vi "Untitled 2.vi"() -> ()   [LabVIEW 2019]
uses:
  <vilib>/OPCUA/controls/OPC UA Client Refnum.ctl
  subVIs/Mode-Ctrl.ctl
  subVIs/CMD-Ctrl.ctl
  <vilib>/OPCUA/controls/Write Variant Request.ctl
  <vilib>/OPCUA/controls/NodeId.ctl
  <vilib>/OPCUA/controls/Write Status.ctl
  <vilib>/OPCUA/client/Multiple Write Variant.vi
  <vilib>/OPCUA/NI OPC UA Client.lvlib
panel:
  out "Control Mode 5":T1
  out "Control Mode 4":T1
  out "Control Mode 3":T1
  out "Control Mode 2":T1
  out "Control Mode":T1
  in  "Reset Alarms UT":bool
  in  "Reset Commands UT":bool
  out "?":T2
  out "?":T2
  in  "Reset Alarms Tube":bool
  in  "Reset Commands Tube":bool
  out "?":T2
  out "?":T2
  in  "Reset Alarms Fork":bool
  in  "Reset Commands Fork":bool
  out "?":T2
  out "?":T2
  in  "Reset Alarms Main2":bool
  in  "Reset Commands Main2":bool
  out "?":T2
  out "?":T2
  in  "Reset Alarms Main1":bool
  in  "Reset Commands Main1":bool
  out "?":T2
  out "?":T2
  in  "error IO":errorcluster
  in  "OPC UA client refnum out":T3
  in  "stop":bool
  # "Main 1"
  # "Main 2"
  # "Fork"
  # "Tube"
  # "UT"
  # "Telescope ShutDown Command"
  # "Alt ShutDown Command"
  # "Az ShutDown Command"
  # "HSB ShutDown Command"
  # "Rotator ShutDown Command"
  # "Adaptor ShutDown Command"
  # "Enclosure ShutDown Command"
  # "MirrorCover ShutDown Command"
  # "Balancin ShutDown Command"
  # "M2 ShutDown Command"
  # "Instrument ShutDown Command"
  # "Control Mode"
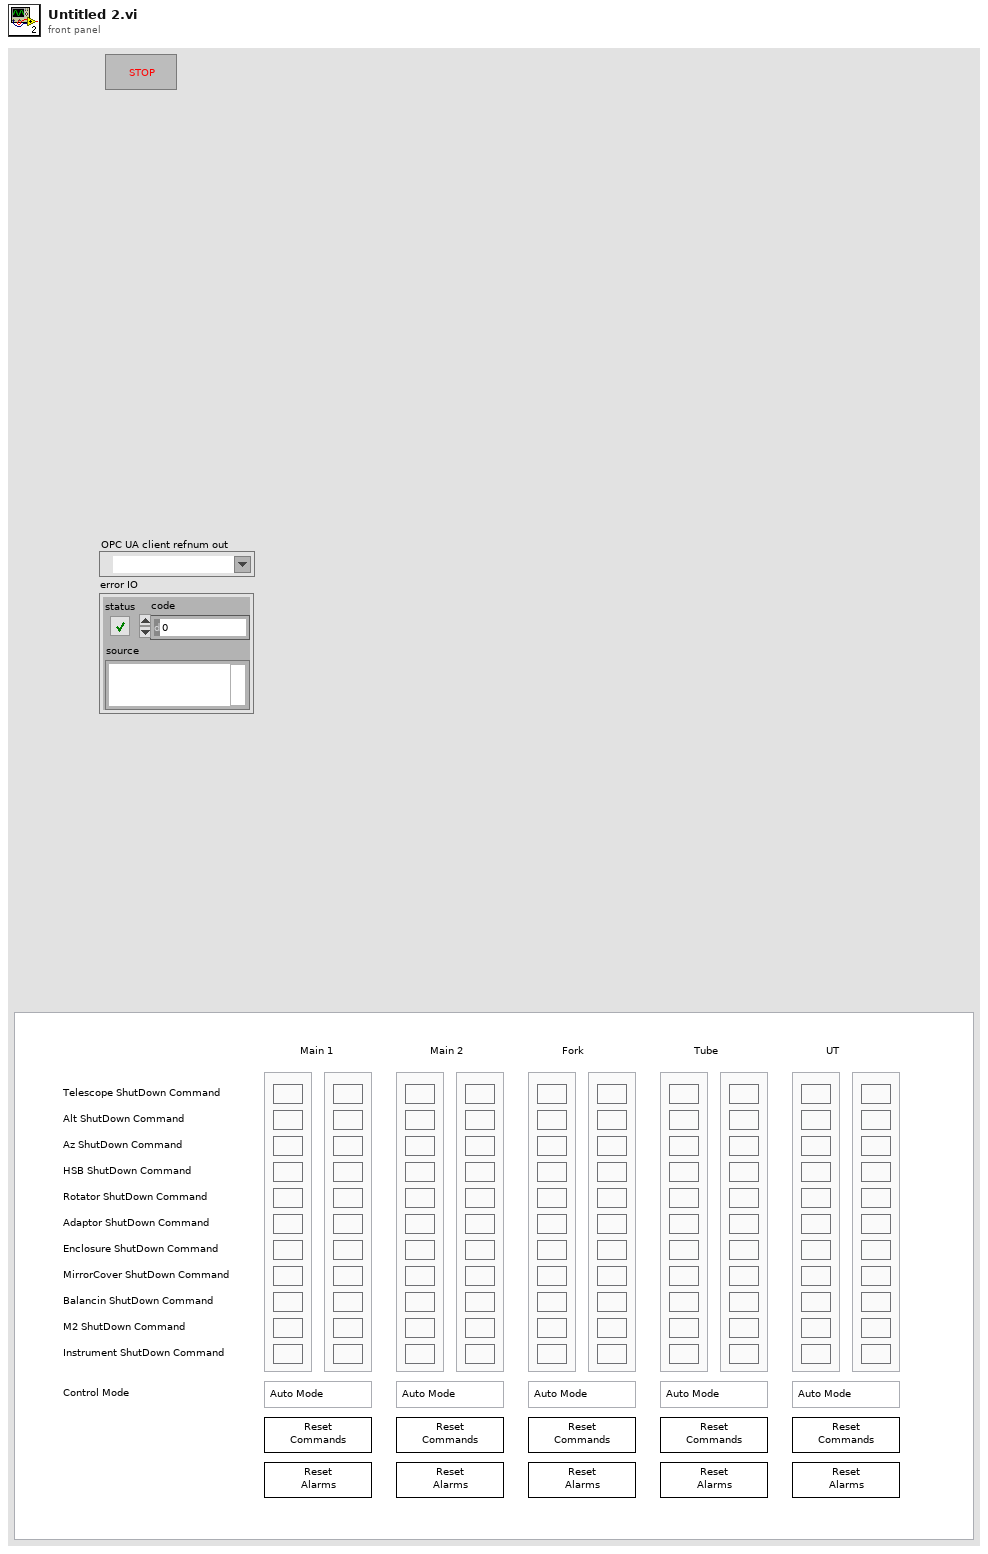
[diagram p1: front panel]
types:
  T1 = typedef "Mode-Ctrl.ctl" = enum16{"Auto Mode", "Maintenance Full Access", "Engineering Mode"}
  T2 = typedef "CMD-Ctrl.ctl" = cluster{"Telescope ShutDown Command":bool, "Alt ShutDown Command":bool, "Az ShutDown Command":bool, "HSB ShutDown Command":bool, "Rotator ShutDown Command":bool, "Adaptor ShutDown Command":bool, "Enclosure ShutDown Command":bool, "MirrorCover ShutDown Command":bool, "Balancing ShutDown Command":bool, "M2 ShutDown Command":bool, "Instrument ShutDown Command":bool}
  T3 = typedef "OPC UA Client Refnum.ctl" = refnum<k21>
  T4 = typedef "Write Variant Request.ctl" = cluster{"node ID":T5, "value":variant, "timestamp (current time)":timestamp, "node status":T6}
  T5 = typedef "NodeId.ctl" = string
  T6 = typedef "Write Status.ctl" = u32
  T7 = typedef "Subscription ID.ctl" = u32
  T8 = typedef "Subscription Data Change.ctl" = cluster{"node ID":T5, " value":variant, "timestamp":timestamp, "data type":T9, "status code":T10}
  T9 = typedef "Data Type.ctl" = u16
  T10 = typedef "OPC UA StatusCode.ctl" = u32
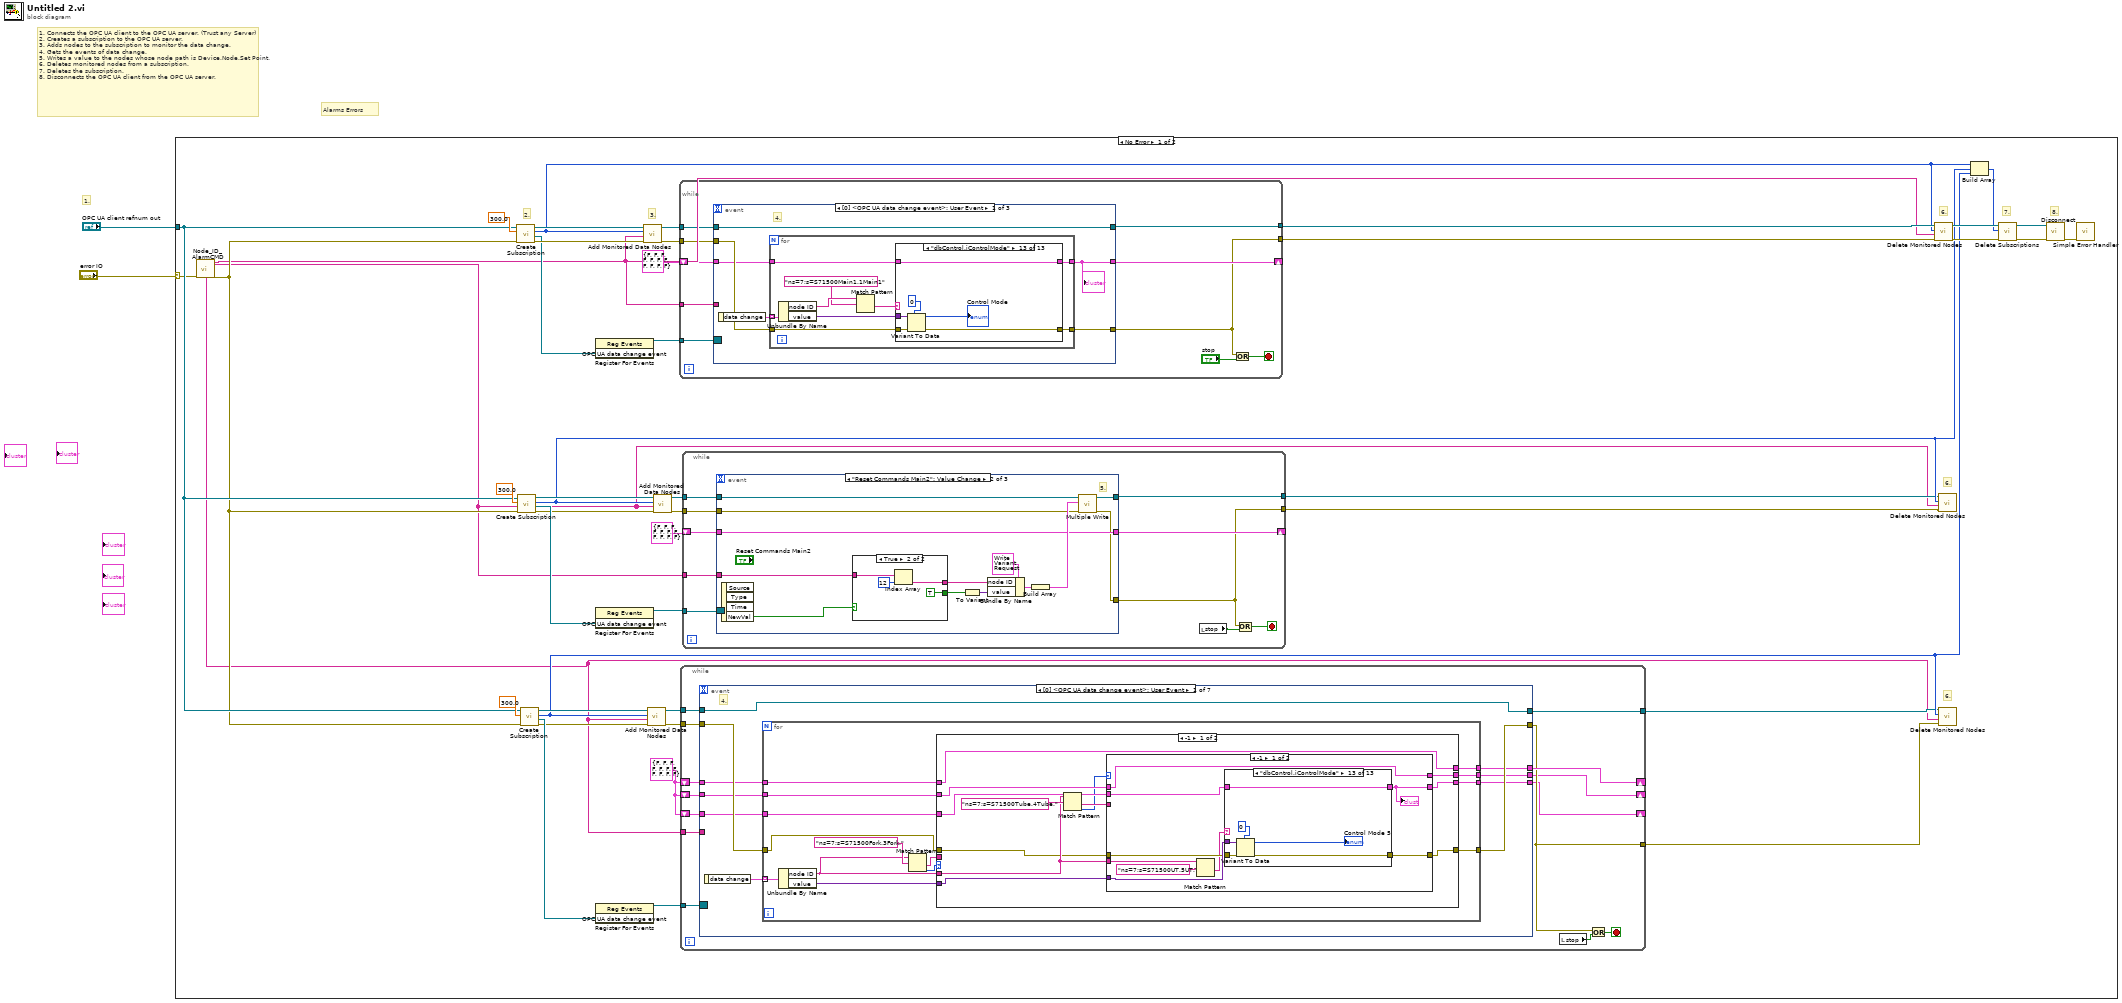
[diagram p0: block diagram]
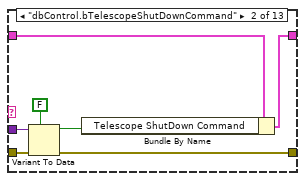
[diagram p3: hidden frame]
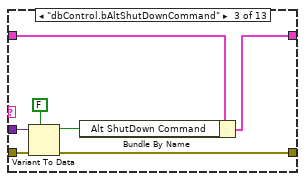
[diagram p4: hidden frame]
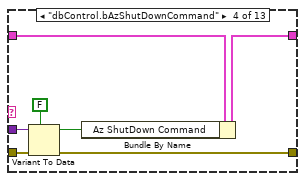
[diagram p5: hidden frame]
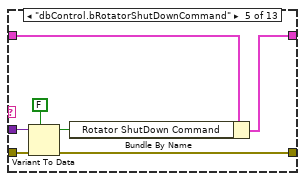
[diagram p6: hidden frame]
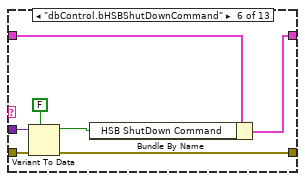
[diagram p7: hidden frame]
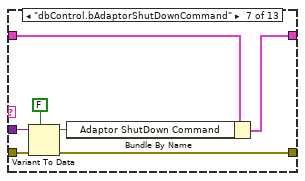
[diagram p8: hidden frame]
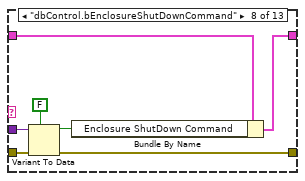
[diagram p9: hidden frame]
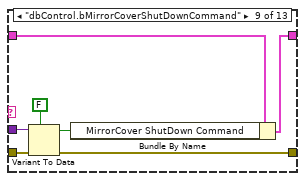
[diagram p10: hidden frame]
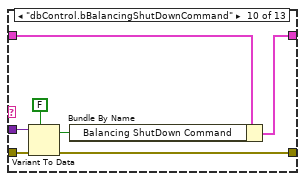
[diagram p11: hidden frame]
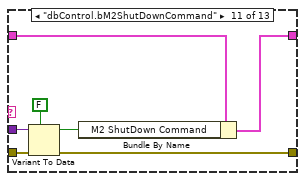
[diagram p12: hidden frame]
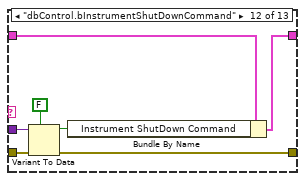
[diagram p13: hidden frame]
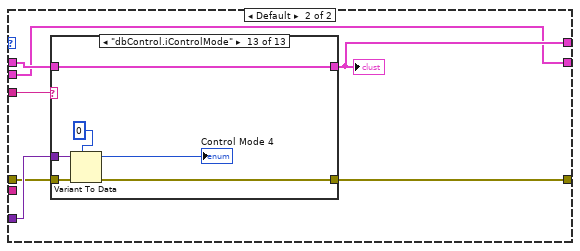
[diagram p14: hidden frame]
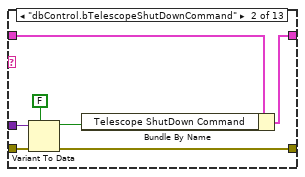
[diagram p16: hidden frame]
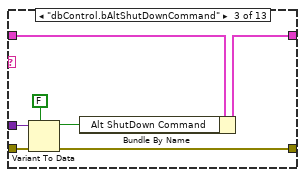
[diagram p17: hidden frame]
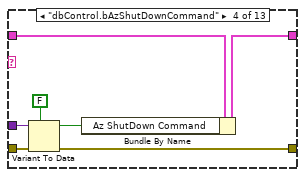
[diagram p18: hidden frame]
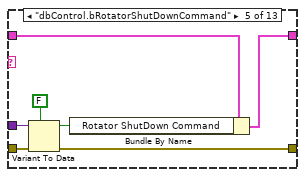
[diagram p19: hidden frame]
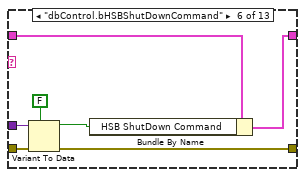
[diagram p20: hidden frame]
diagram:
  # "1."
  # "Alarms Errors"
  # "1. Connects the OPC UA client to the OPC UA server. (Trust any Server) \n2. Creates a subscription to the OPC UA server.\n3. Adds nodes to the subscription to monitor the data change.\n4. Gets the events of data change.\n5. Writes a value to the nodes whose node path is Device.Node.Set Point. \n6. Deletes monitored nodes from a subscription.\n7. Deletes the subscription.\n8. Disconnects the OPC UA client from the OPC UA server."
  n1 = case shown="No Error" "error IO" {
    selector: "error IO" -> [w21 w790]
    tunnel: "OPC UA client refnum out" -> [w26 _]
    frame No Error {
      w5 = T2 {"Telescope ShutDown Command"=FALSE, "Alt ShutDown Command"=FALSE, "Az ShutDown Command"=FALSE, "HSB ShutDown Command"=FALSE, "Rotator ShutDown Command"=FALSE, "Adaptor ShutDown Command"=FALSE, "Enclosure ShutDown Command"=FALSE, "MirrorCover ShutDown Command"=FALSE, "Balancing ShutDown Command"=FALSE, "M2 ShutDown Command"=FALSE, "Instrument ShutDown Command"=FALSE}
      # "6."
      # "6."
      # "7."
      # "8."
      # "6."
      # "3."
      # "2."
      n2 = call "Node_ID_AlarmCMD.vi"("error in"=w21) -> ("appended array"=w3:string[], "Main 1"=w17:string[], "Main 2"=w4:string[], "error out"=w20:errorcluster)  [unwired: 9 in, 6 out]
      n3 = call <vilib>:"Create Subscription.vi"("error in (no error)"=w20, "publishing interval (1000 ms)"=300.0 ("update rate (1000 ms)"), "OPC UA client refnum in"=w26) -> ("error out"=w46:errorcluster, "OPC UA data change event"=w33:refnum<user-event>, "subscription ID out"=w35:T7, "OPC UA client refnum out"=w47:T3)  [unwired: 4 in, 1 out]
      n4 = call <vilib>:"Create Subscription.vi"("error in (no error)"=w20, "publishing interval (1000 ms)"=300.0, "OPC UA client refnum in"=w26) -> ("error out"=w19:errorcluster, "OPC UA data change event"=w29:refnum<user-event>, "subscription ID out"=w28:T7, "OPC UA client refnum out"=w30:T3)  [unwired: 4 in, 1 out]
      n5 = call <vilib>:"Create Subscription.vi"("error in (no error)"=w20, "publishing interval (1000 ms)"=300.0, "OPC UA client refnum in"=w26) -> ("error out"=w23:errorcluster, "OPC UA data change event"=w25:refnum<user-event>, "subscription ID out"=w22:T7, "OPC UA client refnum out"=w24:T3)  [unwired: 4 in, 1 out]
      n6 = register-events(w33) -> (reference out=w45:refnum<event-registration>)  [unwired: 2 in, 1 out]
      n7 = register-events(w29) -> (reference out=w12:refnum<event-registration>)  [unwired: 2 in, 1 out]
      n8 = register-events(w25) -> (reference out=w6:refnum<event-registration>)  [unwired: 2 in, 1 out]
      n9 = call <vilib>:"Add Monitored Data Nodes.vi"("error in (no error)"=w46, "node IDs"=w17, "subscription ID in"=w35, "OPC UA client refnum in"=w47) -> ("error out"=w43:errorcluster, "OPC UA client refnum out"=w44:T3)  [unwired: 4 in, 2 out]
      n10 = call <vilib>:"Add Monitored Data Nodes.vi"("error in (no error)"=w23, "node IDs"=w3, "subscription ID in"=w22, "OPC UA client refnum in"=w24) -> ("error out"=w9:errorcluster, "OPC UA client refnum out"=w10:T3)  [unwired: 4 in, 2 out]
      n11 = call <vilib>:"Add Monitored Data Nodes.vi"("error in (no error)"=w19, "node IDs"=w4, "subscription ID in"=w28, "OPC UA client refnum in"=w30) -> ("error out"=w15:errorcluster, "OPC UA client refnum out"=w16:T3)  [unwired: 4 in, 2 out]
      n12 = while {
        tunnel: w45 -> [w652]
        tunnel: w44 -> [w651]
        tunnel: w43 -> [w650]
        tunnel: [w643] -> w41
        tunnel: [w644] -> w42
        shift-right: [w646] -> _
        shift-left: T2 {"Telescope ShutDown Command"=FALSE, "Alt ShutDown Command"=FALSE, "Az ShutDown Command"=FALSE, "HSB ShutDown Command"=FALSE, "Rotator ShutDown Command"=FALSE, "Adaptor ShutDown Command"=FALSE, "Enclosure ShutDown Command"=FALSE, "MirrorCover ShutDown Command"=FALSE, "Balancing ShutDown Command"=FALSE, "M2 ShutDown Command"=FALSE, "Instrument ShutDown Command"=FALSE} -> [w647]
        tunnel: w17 -> [w645]
        stop <- w649 stop-if-true
        n13 = event shown="[0] <OPC UA data change event>: User Event" {
          selector: w652 -> [_ _ _]
          dyn-events: _ -> [_ _ _]
          timeout: _ -> [_ _ _]
          tunnel: w651 -> [w655 w758 w778]
          tunnel: [w655 w759 w779] -> w644
          tunnel: [w656 w753 w771] -> w643
          tunnel: w650 -> [w657 w754 w772]
          tunnel: w647 -> [w654 w757 w777]
          tunnel: [w653 w757 w777] -> w646
          tunnel: w645 -> [_ w765 w776]
          event User Event {
            # "4."
            n14 = event-data() -> ("data change"=w658:T8[])  [unwired: 1 in]
            n15 = for {
              tunnel: w658 -> [w664] mode=indexing
              tunnel: w657 -> [w666]
              tunnel: [w665] -> w656
              tunnel: w654 -> [w663]
              tunnel: [w662] -> w653
              n16 = Unbundle By Name(w664) -> ("node ID"=w661:T5, "value"=w667:variant)
              n17 = Match Pattern(string=w661, regular expression="ns=7;s=S71500Main1.1Main1" ("string")) -> (after substring=w659:T5)  [unwired: 1 in, 3 out]
              n18 = case shown="\"dbControl.iControlMode\"" w659 {
                tunnel: w667 -> [_ w676 w683 w690 w697 w704 w711 w718 w725 w732 w739 w746 w752]
                tunnel: w666 -> [w669 w674 w681 w688 w695 w702 w709 w716 w723 w730 w737 w744 w751]
                tunnel: [w669 w673 w680 w687 w694 w701 w708 w715 w722 w729 w736 w743 w750] -> w665
                tunnel: w663 -> [w668 w672 w679 w686 w693 w700 w707 w714 w721 w727 w734 w741 w749]
                tunnel: [w668 w671 w678 w685 w692 w699 w706 w713 w720 w726 w733 w740 w749] -> w662
                frame "False", Default {
                }
                frame "dbControl.bTelescopeShutDownCommand" {
                  n19 = Variant To Data(error in=w674, type=FALSE, Variant=w676) -> (data=w670:bool, error out=w673:errorcluster)
                  n20 = Bundle By Name(cluster=w672, "Telescope ShutDown Command"=w670) -> (w671:T2)
                }
                frame "dbControl.bAltShutDownCommand" {
                  n21 = Variant To Data(error in=w681, type=FALSE, Variant=w683) -> (data=w677:bool, error out=w680:errorcluster)
                  n22 = Bundle By Name(cluster=w679, "Alt ShutDown Command"=w677) -> (w678:T2)
                }
                frame "dbControl.bAzShutDownCommand" {
                  n23 = Variant To Data(error in=w688, type=FALSE, Variant=w690) -> (data=w684:bool, error out=w687:errorcluster)
                  n24 = Bundle By Name(cluster=w686, "Az ShutDown Command"=w684) -> (w685:T2)
                }
                frame "dbControl.bRotatorShutDownCommand" {
                  n25 = Variant To Data(error in=w695, type=FALSE, Variant=w697) -> (data=w691:bool, error out=w694:errorcluster)
                  n26 = Bundle By Name(cluster=w693, "Rotator ShutDown Command"=w691) -> (w692:T2)
                }
                frame "dbControl.bHSBShutDownCommand" {
                  n27 = Variant To Data(error in=w702, type=FALSE, Variant=w704) -> (data=w698:bool, error out=w701:errorcluster)
                  n28 = Bundle By Name(cluster=w700, "HSB ShutDown Command"=w698) -> (w699:T2)
                }
                frame "dbControl.bAdaptorShutDownCommand" {
                  n29 = Variant To Data(error in=w709, type=FALSE, Variant=w711) -> (data=w705:bool, error out=w708:errorcluster)
                  n30 = Bundle By Name(cluster=w707, "Adaptor ShutDown Command"=w705) -> (w706:T2)
                }
                frame "dbControl.bEnclosureShutDownCommand" {
                  n31 = Variant To Data(error in=w716, type=FALSE, Variant=w718) -> (data=w712:bool, error out=w715:errorcluster)
                  n32 = Bundle By Name(cluster=w714, "Enclosure ShutDown Command"=w712) -> (w713:T2)
                }
                frame "dbControl.bMirrorCoverShutDownCommand" {
                  n33 = Variant To Data(error in=w723, type=FALSE, Variant=w725) -> (data=w719:bool, error out=w722:errorcluster)
                  n34 = Bundle By Name(cluster=w721, "MirrorCover ShutDown Command"=w719) -> (w720:T2)
                }
                frame "dbControl.bBalancingShutDownCommand" {
                  n35 = Variant To Data(error in=w730, type=FALSE, Variant=w732) -> (data=w728:bool, error out=w729:errorcluster)
                  n36 = Bundle By Name(cluster=w727, "Balancing ShutDown Command"=w728) -> (w726:T2)
                }
                frame "dbControl.bM2ShutDownCommand" {
                  n37 = Variant To Data(error in=w737, type=FALSE, Variant=w739) -> (data=w735:bool, error out=w736:errorcluster)
                  n38 = Bundle By Name(cluster=w734, "M2 ShutDown Command"=w735) -> (w733:T2)
                }
                frame "dbControl.bInstrumentShutDownCommand" {
                  n39 = Variant To Data(error in=w744, type=FALSE, Variant=w746) -> (data=w742:bool, error out=w743:errorcluster)
                  n40 = Bundle By Name(cluster=w741, "Instrument ShutDown Command"=w742) -> (w740:T2)
                }
                frame "dbControl.iControlMode" {
                  n41 = Variant To Data(error in=w751, type=u16 0, Variant=w752) -> (data=→"Control Mode":u16, error out=w750:errorcluster)
                }
              }
            }
            "?" <- w653
          }
          event "Reset Commands Main1": Value Change {
            # "5."
            n42 = event-data() -> ("NewVal"=w755:bool)  [unwired: 1 in, 3 out]
            n43 = case shown="True" w755 {
              tunnel: w765 -> [_ w770]
              tunnel: [_ w769] -> w760
              tunnel: [FALSE TRUE] -> w756
              frame False {
              }
              frame True {
                n44 = Index Array(array=w770, index=12) -> (element=w769:string)
              }
            }
            n45 = To Variant(anything=w756) -> (Variant=w761:variant)
            n46 = Bundle By Name(cluster=T4 {"node ID"="", "value"=variant, "timestamp (current time)"=timestamp(0 s since 1904-01-01), "node status"=0} ("request"), "node ID"=w760, "value"=w761) -> (w764:T4)
            n47 = Build Array(w764) -> (w763:T4[])
            n48 = call-poly <vilib>:"Multiple Write.vi"("error in (no error)"=w754, "requests"=w763, "OPC UA client refnum in"=w758) -> ("error out"=w753:errorcluster, "OPC UA client refnum out"=w759:T3)  [unwired: 5 in, 2 out]
          }
          event "Reset Alarms Main1": Value Change {
            # "5."
            n49 = event-data() -> ("NewVal"=w775:bool)  [unwired: 1 in, 3 out]
            n50 = case shown="True" w775 {
              tunnel: w776 -> [_ w788]
              tunnel: [_ w787] -> w774
              tunnel: [FALSE TRUE] -> w773
              frame False {
              }
              frame True {
                n51 = Index Array(array=w788, index=13) -> (element=w787:string)
              }
            }
            n52 = To Variant(anything=w773) -> (Variant=w780:variant)
            n53 = Bundle By Name(cluster=T4 {"node ID"="", "value"=variant, "timestamp (current time)"=timestamp(0 s since 1904-01-01), "node status"=0} ("request"), "node ID"=w774, "value"=w780) -> (w783:T4)
            n54 = Build Array(w783) -> (w782:T4[])
            n55 = call-poly <vilib>:"Multiple Write.vi"("error in (no error)"=w772, "requests"=w782, "OPC UA client refnum in"=w778) -> ("error out"=w771:errorcluster, "OPC UA client refnum out"=w779:T3)  [unwired: 5 in, 2 out]
          }
        }
        n56 = Or(x=w643, y="stop") -> (x .or. y?=w649:bool)
      }
      n57 = while {
        tunnel: w6 -> [w61]
        tunnel: w10 -> [w60]
        tunnel: w9 -> [w59]
        tunnel: [w53] -> w7
        tunnel: [w54] -> w8
        shift-right: [w56] -> _
        shift-left: w5 -> [w57]
        tunnel: w3 -> [w55]
        shift-right: [w50] -> _
        shift-left: w5 -> [w51]
        shift-right: [w48] -> _
        shift-left: w5 -> [w49]
        stop <- w58 stop-if-true
        n58 = event shown="[0] <OPC UA data change event>: User Event" {
          selector: w61 -> [_ _ _ _ _ _ _]
          dyn-events: _ -> [_ _ _ _ _ _ _]
          timeout: _ -> [_ _ _ _ _ _ _]
          tunnel: w60 -> [w68 w384 w404 w424 w444 w464 w484]
          tunnel: [w68 w385 w405 w425 w445 w465 w485] -> w54
          tunnel: [w69 w379 w399 w419 w439 w459 w479] -> w53
          tunnel: w59 -> [w70 w380 w400 w420 w440 w460 w480]
          tunnel: w57 -> [w67 w383 w403 w423 w443 w463 w483]
          tunnel: [w66 w383 w403 w423 w443 w463 w483] -> w56
          tunnel: w55 -> [_ w391 w411 w431 w451 w471 w491]
          tunnel: w51 -> [w65 w378 w398 w418 w438 w458 w478]
          tunnel: [w64 w378 w398 w418 w438 w458 w478] -> w50
          tunnel: w49 -> [w63 w377 w397 w417 w437 w457 w477]
          tunnel: [w62 w377 w397 w417 w437 w457 w477] -> w48
          event User Event {
            # "4."
            n59 = event-data() -> ("data change"=w71:T8[])  [unwired: 1 in]
            n60 = for {
              tunnel: w71 -> [w82] mode=indexing
              tunnel: w70 -> [w84]
              tunnel: [w83] -> w69
              tunnel: w67 -> [w81]
              tunnel: [w80] -> w66
              tunnel: w65 -> [w75]
              tunnel: [w74] -> w64
              tunnel: w63 -> [w73]
              tunnel: [w72] -> w62
              n61 = Unbundle By Name(w82) -> ("node ID"=w76:T5, "value"=w85:variant)
              n62 = Match Pattern(string=w76, regular expression="ns=7;s=S71500Fork.3Fork." ("string")) -> (after substring=w78:T5, offset past match=w77:i32)  [unwired: 1 in, 2 out]
              n63 = case shown="-1" w77 {
                tunnel: w85 -> [w94 w291]
                tunnel: w84 -> [w87 w290]
                tunnel: [w91 w289] -> w83
                tunnel: w81 -> [w86 w288]
                tunnel: [w86 w286] -> w80
                tunnel: w78 -> [_ w287]
                tunnel: w76 -> [w96 _]
                tunnel: w75 -> [w93 w285]
                tunnel: [w92 w285] -> w74
                tunnel: w73 -> [w90 w284]
                tunnel: [w89 w284] -> w72
                frame -1 {
                  n64 = Match Pattern(string=w96, regular expression="ns=7;s=S71500Tube.4Tube." ("string")) -> (after substring=w95:T5, offset past match=w88:i32)  [unwired: 1 in, 2 out]
                  n65 = case shown="-1" w88 {
                    tunnel: w96 -> [w104 _]
                    tunnel: w95 -> [_ w193]
                    tunnel: w94 -> [w103 w198]
                    tunnel: w87 -> [w102 w197]
                    tunnel: w93 -> [w106 w196]
                    tunnel: [w106 w195] -> w92
                    tunnel: [w101 w192] -> w91
                    tunnel: w90 -> [w99 w194]
                    tunnel: [w98 w194] -> w89
                    frame -1 {
                      n66 = Match Pattern(string=w104, regular expression="ns=7;s=S71500UT.5UT." ("string")) -> (after substring=w100:T5)  [unwired: 1 in, 3 out]
                      n67 = case shown="\"dbControl.iControlMode\"" w100 {
                        tunnel: w103 -> [_ w115 w122 w129 w136 w143 w150 w157 w164 w171 w178 w185 w191]
                        tunnel: w102 -> [w108 w113 w120 w127 w134 w141 w148 w155 w162 w169 w176 w183 w190]
                        tunnel: [w108 w112 w119 w126 w133 w140 w147 w154 w161 w168 w175 w182 w189] -> w101
                        tunnel: w99 -> [w107 w111 w118 w125 w132 w139 w146 w153 w160 w166 w173 w180 w188]
                        tunnel: [w107 w110 w117 w124 w131 w138 w145 w152 w159 w165 w172 w179 w188] -> w98
                        frame "False", Default {
                        }
                        frame "dbControl.bTelescopeShutDownCommand" {
                          n68 = Variant To Data(error in=w113, type=FALSE, Variant=w115) -> (data=w109:bool, error out=w112:errorcluster)
                          n69 = Bundle By Name(cluster=w111, "Telescope ShutDown Command"=w109) -> (w110:T2)
                        }
                        frame "dbControl.bAltShutDownCommand" {
                          n70 = Variant To Data(error in=w120, type=FALSE, Variant=w122) -> (data=w116:bool, error out=w119:errorcluster)
                          n71 = Bundle By Name(cluster=w118, "Alt ShutDown Command"=w116) -> (w117:T2)
                        }
                        frame "dbControl.bAzShutDownCommand" {
                          n72 = Variant To Data(error in=w127, type=FALSE, Variant=w129) -> (data=w123:bool, error out=w126:errorcluster)
                          n73 = Bundle By Name(cluster=w125, "Az ShutDown Command"=w123) -> (w124:T2)
                        }
                        frame "dbControl.bRotatorShutDownCommand" {
                          n74 = Variant To Data(error in=w134, type=FALSE, Variant=w136) -> (data=w130:bool, error out=w133:errorcluster)
                          n75 = Bundle By Name(cluster=w132, "Rotator ShutDown Command"=w130) -> (w131:T2)
                        }
                        frame "dbControl.bHSBShutDownCommand" {
                          n76 = Variant To Data(error in=w141, type=FALSE, Variant=w143) -> (data=w137:bool, error out=w140:errorcluster)
                          n77 = Bundle By Name(cluster=w139, "HSB ShutDown Command"=w137) -> (w138:T2)
                        }
                        frame "dbControl.bAdaptorShutDownCommand" {
                          n78 = Variant To Data(error in=w148, type=FALSE, Variant=w150) -> (data=w144:bool, error out=w147:errorcluster)
                          n79 = Bundle By Name(cluster=w146, "Adaptor ShutDown Command"=w144) -> (w145:T2)
                        }
                        frame "dbControl.bEnclosureShutDownCommand" {
                          n80 = Variant To Data(error in=w155, type=FALSE, Variant=w157) -> (data=w151:bool, error out=w154:errorcluster)
                          n81 = Bundle By Name(cluster=w153, "Enclosure ShutDown Command"=w151) -> (w152:T2)
                        }
                        frame "dbControl.bMirrorCoverShutDownCommand" {
                          n82 = Variant To Data(error in=w162, type=FALSE, Variant=w164) -> (data=w158:bool, error out=w161:errorcluster)
                          n83 = Bundle By Name(cluster=w160, "MirrorCover ShutDown Command"=w158) -> (w159:T2)
                        }
                        frame "dbControl.bBalancingShutDownCommand" {
                          n84 = Variant To Data(error in=w169, type=FALSE, Variant=w171) -> (data=w167:bool, error out=w168:errorcluster)
                          n85 = Bundle By Name(cluster=w166, "Balancing ShutDown Command"=w167) -> (w165:T2)
                        }
                        frame "dbControl.bM2ShutDownCommand" {
                          n86 = Variant To Data(error in=w176, type=FALSE, Variant=w178) -> (data=w174:bool, error out=w175:errorcluster)
                          n87 = Bundle By Name(cluster=w173, "M2 ShutDown Command"=w174) -> (w172:T2)
                        }
                        frame "dbControl.bInstrumentShutDownCommand" {
                          n88 = Variant To Data(error in=w183, type=FALSE, Variant=w185) -> (data=w181:bool, error out=w182:errorcluster)
                          n89 = Bundle By Name(cluster=w180, "Instrument ShutDown Command"=w181) -> (w179:T2)
                        }
                        frame "dbControl.iControlMode" {
                          n90 = Variant To Data(error in=w190, type=u16 0, Variant=w191) -> (data=→"Control Mode 5":u16, error out=w189:errorcluster)
                        }
                      }
                      "?" <- w98
                    }
                    frame Default {
                      n91 = case shown="\"dbControl.iControlMode\"" w193 {
                        tunnel: w198 -> [_ w207 w214 w221 w228 w235 w242 w249 w256 w263 w270 w277 w283]
                        tunnel: w197 -> [w200 w205 w212 w219 w226 w233 w240 w247 w254 w261 w268 w275 w282]
                        tunnel: [w200 w204 w211 w218 w225 w232 w239 w246 w253 w260 w267 w274 w281] -> w192
                        tunnel: w196 -> [w199 w203 w210 w217 w224 w231 w238 w245 w252 w258 w265 w272 w280]
                        tunnel: [w199 w202 w209 w216 w223 w230 w237 w244 w251 w257 w264 w271 w280] -> w195
                        frame "False", Default {
                        }
                        frame "dbControl.bTelescopeShutDownCommand" {
                          n92 = Variant To Data(error in=w205, type=FALSE, Variant=w207) -> (data=w201:bool, error out=w204:errorcluster)
                          n93 = Bundle By Name(cluster=w203, "Telescope ShutDown Command"=w201) -> (w202:T2)
                        }
                        frame "dbControl.bAltShutDownCommand" {
                          n94 = Variant To Data(error in=w212, type=FALSE, Variant=w214) -> (data=w208:bool, error out=w211:errorcluster)
                          n95 = Bundle By Name(cluster=w210, "Alt ShutDown Command"=w208) -> (w209:T2)
                        }
                        frame "dbControl.bAzShutDownCommand" {
                          n96 = Variant To Data(error in=w219, type=FALSE, Variant=w221) -> (data=w215:bool, error out=w218:errorcluster)
                          n97 = Bundle By Name(cluster=w217, "Az ShutDown Command"=w215) -> (w216:T2)
                        }
                        frame "dbControl.bRotatorShutDownCommand" {
                          n98 = Variant To Data(error in=w226, type=FALSE, Variant=w228) -> (data=w222:bool, error out=w225:errorcluster)
                          n99 = Bundle By Name(cluster=w224, "Rotator ShutDown Command"=w222) -> (w223:T2)
                        }
                        frame "dbControl.bHSBShutDownCommand" {
                          n100 = Variant To Data(error in=w233, type=FALSE, Variant=w235) -> (data=w229:bool, error out=w232:errorcluster)
                          n101 = Bundle By Name(cluster=w231, "HSB ShutDown Command"=w229) -> (w230:T2)
                        }
                        frame "dbControl.bAdaptorShutDownCommand" {
                          n102 = Variant To Data(error in=w240, type=FALSE, Variant=w242) -> (data=w236:bool, error out=w239:errorcluster)
                          n103 = Bundle By Name(cluster=w238, "Adaptor ShutDown Command"=w236) -> (w237:T2)
                        }
                        frame "dbControl.bEnclosureShutDownCommand" {
                          n104 = Variant To Data(error in=w247, type=FALSE, Variant=w249) -> (data=w243:bool, error out=w246:errorcluster)
                          n105 = Bundle By Name(cluster=w245, "Enclosure ShutDown Command"=w243) -> (w244:T2)
                        }
                        frame "dbControl.bMirrorCoverShutDownCommand" {
                          n106 = Variant To Data(error in=w254, type=FALSE, Variant=w256) -> (data=w250:bool, error out=w253:errorcluster)
                          n107 = Bundle By Name(cluster=w252, "MirrorCover ShutDown Command"=w250) -> (w251:T2)
                        }
                        frame "dbControl.bBalancingShutDownCommand" {
                          n108 = Variant To Data(error in=w261, type=FALSE, Variant=w263) -> (data=w259:bool, error out=w260:errorcluster)
                          n109 = Bundle By Name(cluster=w258, "Balancing ShutDown Command"=w259) -> (w257:T2)
                        }
                        frame "dbControl.bM2ShutDownCommand" {
                          n110 = Variant To Data(error in=w268, type=FALSE, Variant=w270) -> (data=w266:bool, error out=w267:errorcluster)
                          n111 = Bundle By Name(cluster=w265, "M2 ShutDown Command"=w266) -> (w264:T2)
                        }
                        frame "dbControl.bInstrumentShutDownCommand" {
                          n112 = Variant To Data(error in=w275, type=FALSE, Variant=w277) -> (data=w273:bool, error out=w274:errorcluster)
                          n113 = Bundle By Name(cluster=w272, "Instrument ShutDown Command"=w273) -> (w271:T2)
                        }
                        frame "dbControl.iControlMode" {
                          n114 = Variant To Data(error in=w282, type=u16 0, Variant=w283) -> (data=→"Control Mode 4":u16, error out=w281:errorcluster)
                        }
                      }
                      "?" <- w195
                    }
                  }
                }
                frame Default {
                  n115 = case shown="\"dbControl.iControlMode\"" w287 {
                    tunnel: w291 -> [_ w300 w307 w314 w321 w328 w335 w342 w349 w356 w363 w370 w376]
                    tunnel: w290 -> [w293 w298 w305 w312 w319 w326 w333 w340 w347 w354 w361 w368 w375]
                    tunnel: [w293 w297 w304 w311 w318 w325 w332 w339 w346 w353 w360 w367 w374] -> w289
                    tunnel: w288 -> [w292 w296 w303 w310 w317 w324 w331 w338 w345 w351 w358 w365 w373]
                    tunnel: [w292 w295 w302 w309 w316 w323 w330 w337 w344 w350 w357 w364 w373] -> w286
                    frame "False", Default {
                    }
                    frame "dbControl.bTelescopeShutDownCommand" {
                      n116 = Variant To Data(error in=w298, type=FALSE, Variant=w300) -> (data=w294:bool, error out=w297:errorcluster)
                      n117 = Bundle By Name(cluster=w296, "Telescope ShutDown Command"=w294) -> (w295:T2)
                    }
                    frame "dbControl.bAltShutDownCommand" {
                      n118 = Variant To Data(error in=w305, type=FALSE, Variant=w307) -> (data=w301:bool, error out=w304:errorcluster)
                      n119 = Bundle By Name(cluster=w303, "Alt ShutDown Command"=w301) -> (w302:T2)
                    }
                    frame "dbControl.bAzShutDownCommand" {
                      n120 = Variant To Data(error in=w312, type=FALSE, Variant=w314) -> (data=w308:bool, error out=w311:errorcluster)
                      n121 = Bundle By Name(cluster=w310, "Az ShutDown Command"=w308) -> (w309:T2)
                    }
                    frame "dbControl.bRotatorShutDownCommand" {
                      n122 = Variant To Data(error in=w319, type=FALSE, Variant=w321) -> (data=w315:bool, error out=w318:errorcluster)
                      n123 = Bundle By Name(cluster=w317, "Rotator ShutDown Command"=w315) -> (w316:T2)
                    }
                    frame "dbControl.bHSBShutDownCommand" {
                      n124 = Variant To Data(error in=w326, type=FALSE, Variant=w328) -> (data=w322:bool, error out=w325:errorcluster)
                      n125 = Bundle By Name(cluster=w324, "HSB ShutDown Command"=w322) -> (w323:T2)
                    }
                    frame "dbControl.bAdaptorShutDownCommand" {
                      n126 = Variant To Data(error in=w333, type=FALSE, Variant=w335) -> (data=w329:bool, error out=w332:errorcluster)
                      n127 = Bundle By Name(cluster=w331, "Adaptor ShutDown Command"=w329) -> (w330:T2)
                    }
                    frame "dbControl.bEnclosureShutDownCommand" {
                      n128 = Variant To Data(error in=w340, type=FALSE, Variant=w342) -> (data=w336:bool, error out=w339:errorcluster)
                      n129 = Bundle By Name(cluster=w338, "Enclosure ShutDown Command"=w336) -> (w337:T2)
                    }
                    frame "dbControl.bMirrorCoverShutDownCommand" {
                      n130 = Variant To Data(error in=w347, type=FALSE, Variant=w349) -> (data=w343:bool, error out=w346:errorcluster)
                      n131 = Bundle By Name(cluster=w345, "MirrorCover ShutDown Command"=w343) -> (w344:T2)
                    }
                    frame "dbControl.bBalancingShutDownCommand" {
                      n132 = Variant To Data(error in=w354, type=FALSE, Variant=w356) -> (data=w352:bool, error out=w353:errorcluster)
                      n133 = Bundle By Name(cluster=w351, "Balancing ShutDown Command"=w352) -> (w350:T2)
                    }
                    frame "dbControl.bM2ShutDownCommand" {
                      n134 = Variant To Data(error in=w361, type=FALSE, Variant=w363) -> (data=w359:bool, error out=w360:errorcluster)
                      n135 = Bundle By Name(cluster=w358, "M2 ShutDown Command"=w359) -> (w357:T2)
                    }
                    frame "dbControl.bInstrumentShutDownCommand" {
                      n136 = Variant To Data(error in=w368, type=FALSE, Variant=w370) -> (data=w366:bool, error out=w367:errorcluster)
                      n137 = Bundle By Name(cluster=w365, "Instrument ShutDown Command"=w366) -> (w364:T2)
                    }
                    frame "dbControl.iControlMode" {
                      n138 = Variant To Data(error in=w375, type=u16 0, Variant=w376) -> (data=→"Control Mode 3":u16, error out=w374:errorcluster)
                    }
                  }
                  "?" <- w286
                }
              }
            }
          }
          event "Reset Commands Fork": Value Change {
            # "5."
            n139 = event-data() -> ("NewVal"=w381:bool)  [unwired: 1 in, 3 out]
            n140 = case shown="True" w381 {
              tunnel: w391 -> [_ w396]
              tunnel: [_ w395] -> w386
              tunnel: [FALSE TRUE] -> w382
              frame False {
              }
              frame True {
                n141 = Index Array(array=w396, index=12) -> (element=w395:string)
              }
            }
            n142 = To Variant(anything=w382) -> (Variant=w387:variant)
            n143 = Bundle By Name(cluster=T4 {"node ID"="", "value"=variant, "timestamp (current time)"=timestamp(0 s since 1904-01-01), "node status"=0} ("request"), "node ID"=w386, "value"=w387) -> (w390:T4)
            n144 = Build Array(w390) -> (w389:T4[])
            n145 = call-poly <vilib>:"Multiple Write.vi"("error in (no error)"=w380, "requests"=w389, "OPC UA client refnum in"=w384) -> ("error out"=w379:errorcluster, "OPC UA client refnum out"=w385:T3)  [unwired: 5 in, 2 out]
          }
          event "Reset Alarms Fork": Value Change {
            # "5."
            n146 = event-data() -> ("NewVal"=w401:bool)  [unwired: 1 in, 3 out]
            n147 = case shown="True" w401 {
              tunnel: w411 -> [_ w416]
              tunnel: [_ w415] -> w406
              tunnel: [FALSE TRUE] -> w402
              frame False {
              }
              frame True {
                n148 = Index Array(array=w416, index=12) -> (element=w415:string)
              }
            }
            n149 = To Variant(anything=w402) -> (Variant=w407:variant)
            n150 = Bundle By Name(cluster=T4 {"node ID"="", "value"=variant, "timestamp (current time)"=timestamp(0 s since 1904-01-01), "node status"=0} ("request"), "node ID"=w406, "value"=w407) -> (w410:T4)
            n151 = Build Array(w410) -> (w409:T4[])
            n152 = call-poly <vilib>:"Multiple Write.vi"("error in (no error)"=w400, "requests"=w409, "OPC UA client refnum in"=w404) -> ("error out"=w399:errorcluster, "OPC UA client refnum out"=w405:T3)  [unwired: 5 in, 2 out]
          }
          event "Reset Commands Tube": Value Change {
            # "5."
            n153 = event-data() -> ("NewVal"=w421:bool)  [unwired: 1 in, 3 out]
            n154 = case shown="True" w421 {
              tunnel: w431 -> [_ w436]
              tunnel: [_ w435] -> w426
              tunnel: [FALSE TRUE] -> w422
              frame False {
              }
              frame True {
                n155 = Index Array(array=w436, index=12) -> (element=w435:string)
              }
            }
            n156 = To Variant(anything=w422) -> (Variant=w427:variant)
            n157 = Bundle By Name(cluster=T4 {"node ID"="", "value"=variant, "timestamp (current time)"=timestamp(0 s since 1904-01-01), "node status"=0} ("request"), "node ID"=w426, "value"=w427) -> (w430:T4)
            n158 = Build Array(w430) -> (w429:T4[])
            n159 = call-poly <vilib>:"Multiple Write.vi"("error in (no error)"=w420, "requests"=w429, "OPC UA client refnum in"=w424) -> ("error out"=w419:errorcluster, "OPC UA client refnum out"=w425:T3)  [unwired: 5 in, 2 out]
          }
          event "Reset Alarms Tube": Value Change {
            # "5."
            n160 = event-data() -> ("NewVal"=w441:bool)  [unwired: 1 in, 3 out]
            n161 = case shown="True" w441 {
              tunnel: w451 -> [_ w456]
              tunnel: [_ w455] -> w446
              tunnel: [FALSE TRUE] -> w442
              frame False {
              }
              frame True {
                n162 = Index Array(array=w456, index=12) -> (element=w455:string)
              }
            }
            n163 = To Variant(anything=w442) -> (Variant=w447:variant)
            n164 = Bundle By Name(cluster=T4 {"node ID"="", "value"=variant, "timestamp (current time)"=timestamp(0 s since 1904-01-01), "node status"=0} ("request"), "node ID"=w446, "value"=w447) -> (w450:T4)
            n165 = Build Array(w450) -> (w449:T4[])
            n166 = call-poly <vilib>:"Multiple Write.vi"("error in (no error)"=w440, "requests"=w449, "OPC UA client refnum in"=w444) -> ("error out"=w439:errorcluster, "OPC UA client refnum out"=w445:T3)  [unwired: 5 in, 2 out]
          }
          event "Reset Commands UT": Value Change {
            # "5."
            n167 = event-data() -> ("NewVal"=w461:bool)  [unwired: 1 in, 3 out]
            n168 = case shown="True" w461 {
              tunnel: w471 -> [_ w476]
              tunnel: [_ w475] -> w466
              tunnel: [FALSE TRUE] -> w462
              frame False {
              }
              frame True {
                n169 = Index Array(array=w476, index=12) -> (element=w475:string)
              }
            }
            n170 = To Variant(anything=w462) -> (Variant=w467:variant)
            n171 = Bundle By Name(cluster=T4 {"node ID"="", "value"=variant, "timestamp (current time)"=timestamp(0 s since 1904-01-01), "node status"=0} ("request"), "node ID"=w466, "value"=w467) -> (w470:T4)
            n172 = Build Array(w470) -> (w469:T4[])
            n173 = call-poly <vilib>:"Multiple Write.vi"("error in (no error)"=w460, "requests"=w469, "OPC UA client refnum in"=w464) -> ("error out"=w459:errorcluster, "OPC UA client refnum out"=w465:T3)  [unwired: 5 in, 2 out]
          }
          event "Reset Alarms UT": Value Change {
            # "5."
            n174 = event-data() -> ("NewVal"=w481:bool)  [unwired: 1 in, 3 out]
            n175 = case shown="True" w481 {
              tunnel: w491 -> [_ w496]
              tunnel: [_ w495] -> w486
              tunnel: [FALSE TRUE] -> w482
              frame False {
              }
              frame True {
                n176 = Index Array(array=w496, index=12) -> (element=w495:string)
              }
            }
            n177 = To Variant(anything=w482) -> (Variant=w487:variant)
            n178 = Bundle By Name(cluster=T4 {"node ID"="", "value"=variant, "timestamp (current time)"=timestamp(0 s since 1904-01-01), "node status"=0} ("request"), "node ID"=w486, "value"=w487) -> (w490:T4)
            n179 = Build Array(w490) -> (w489:T4[])
            n180 = call-poly <vilib>:"Multiple Write.vi"("error in (no error)"=w480, "requests"=w489, "OPC UA client refnum in"=w484) -> ("error out"=w479:errorcluster, "OPC UA client refnum out"=w485:T3)  [unwired: 5 in, 2 out]
          }
        }
        n181 = local read "stop"() -> (w52:bool)
        n182 = Or(x=w53, y=w52) -> (x .or. y?=w58:bool)
      }
      n183 = while {
        tunnel: w12 -> [w506]
        tunnel: w16 -> [w505]
        tunnel: w15 -> [w504]
        tunnel: [w498] -> w13
        tunnel: [w499] -> w14
        shift-right: [w501] -> _
        shift-left: T2 {"Telescope ShutDown Command"=FALSE, "Alt ShutDown Command"=FALSE, "Az ShutDown Command"=FALSE, "HSB ShutDown Command"=FALSE, "Rotator ShutDown Command"=FALSE, "Adaptor ShutDown Command"=FALSE, "Enclosure ShutDown Command"=FALSE, "MirrorCover ShutDown Command"=FALSE, "Balancing ShutDown Command"=FALSE, "M2 ShutDown Command"=FALSE, "Instrument ShutDown Command"=FALSE} -> [w502]
        tunnel: w4 -> [w500]
        stop <- w503 stop-if-true
        n184 = event shown="[1] \"Reset Commands Main2\": Value Change" {
          selector: w506 -> [_ _ _]
          dyn-events: _ -> [_ _ _]
          timeout: _ -> [_ _ _]
          tunnel: w505 -> [w509 w612 w632]
          tunnel: [w509 w613 w633] -> w499
          tunnel: [w510 w607 w625] -> w498
          tunnel: w504 -> [w511 w608 w626]
          tunnel: w502 -> [w508 w611 w631]
          tunnel: [w507 w611 w631] -> w501
          tunnel: w500 -> [_ w619 w630]
          event User Event {
            # "4."
            n185 = event-data() -> ("data change"=w512:T8[])  [unwired: 1 in]
            n186 = for {
              tunnel: w512 -> [w518] mode=indexing
              tunnel: w511 -> [w520]
              tunnel: [w519] -> w510
              tunnel: w508 -> [w517]
              tunnel: [w516] -> w507
              n187 = Unbundle By Name(w518) -> ("node ID"=w515:T5, "value"=w521:variant)
              n188 = Match Pattern(string=w515, regular expression="ns=7;s=S71500Main2.2Main2." ("string")) -> (after substring=w513:T5)  [unwired: 1 in, 3 out]
              n189 = case shown="\"False\", Default" w513 {
                tunnel: w521 -> [_ w530 w537 w544 w551 w558 w565 w572 w579 w586 w593 w600 w606]
                tunnel: w520 -> [w523 w528 w535 w542 w549 w556 w563 w570 w577 w584 w591 w598 w605]
                tunnel: [w523 w527 w534 w541 w548 w555 w562 w569 w576 w583 w590 w597 w604] -> w519
                tunnel: w517 -> [w522 w526 w533 w540 w547 w554 w561 w568 w575 w581 w588 w595 w603]
                tunnel: [w522 w525 w532 w539 w546 w553 w560 w567 w574 w580 w587 w594 w603] -> w516
                frame "False", Default {
                }
                frame "dbControl.bTelescopeShutDownCommand" {
                  n190 = Variant To Data(error in=w528, type=FALSE, Variant=w530) -> (data=w524:bool, error out=w527:errorcluster)
                  n191 = Bundle By Name(cluster=w526, "Telescope ShutDown Command"=w524) -> (w525:T2)
                }
                frame "dbControl.bAltShutDownCommand" {
                  n192 = Variant To Data(error in=w535, type=FALSE, Variant=w537) -> (data=w531:bool, error out=w534:errorcluster)
                  n193 = Bundle By Name(cluster=w533, "Alt ShutDown Command"=w531) -> (w532:T2)
                }
                frame "dbControl.bAzShutDownCommand" {
                  n194 = Variant To Data(error in=w542, type=FALSE, Variant=w544) -> (data=w538:bool, error out=w541:errorcluster)
                  n195 = Bundle By Name(cluster=w540, "Az ShutDown Command"=w538) -> (w539:T2)
                }
                frame "dbControl.bRotatorShutDownCommand" {
                  n196 = Variant To Data(error in=w549, type=FALSE, Variant=w551) -> (data=w545:bool, error out=w548:errorcluster)
                  n197 = Bundle By Name(cluster=w547, "Rotator ShutDown Command"=w545) -> (w546:T2)
                }
                frame "dbControl.bHSBShutDownCommand" {
                  n198 = Variant To Data(error in=w556, type=FALSE, Variant=w558) -> (data=w552:bool, error out=w555:errorcluster)
                  n199 = Bundle By Name(cluster=w554, "HSB ShutDown Command"=w552) -> (w553:T2)
                }
                frame "dbControl.bAdaptorShutDownCommand" {
                  n200 = Variant To Data(error in=w563, type=FALSE, Variant=w565) -> (data=w559:bool, error out=w562:errorcluster)
                  n201 = Bundle By Name(cluster=w561, "Adaptor ShutDown Command"=w559) -> (w560:T2)
                }
                frame "dbControl.bEnclosureShutDownCommand" {
                  n202 = Variant To Data(error in=w570, type=FALSE, Variant=w572) -> (data=w566:bool, error out=w569:errorcluster)
                  n203 = Bundle By Name(cluster=w568, "Enclosure ShutDown Command"=w566) -> (w567:T2)
                }
                frame "dbControl.bMirrorCoverShutDownCommand" {
                  n204 = Variant To Data(error in=w577, type=FALSE, Variant=w579) -> (data=w573:bool, error out=w576:errorcluster)
                  n205 = Bundle By Name(cluster=w575, "MirrorCover ShutDown Command"=w573) -> (w574:T2)
                }
                frame "dbControl.bBalancingShutDownCommand" {
                  n206 = Variant To Data(error in=w584, type=FALSE, Variant=w586) -> (data=w582:bool, error out=w583:errorcluster)
                  n207 = Bundle By Name(cluster=w581, "Balancing ShutDown Command"=w582) -> (w580:T2)
                }
                frame "dbControl.bM2ShutDownCommand" {
                  n208 = Variant To Data(error in=w591, type=FALSE, Variant=w593) -> (data=w589:bool, error out=w590:errorcluster)
                  n209 = Bundle By Name(cluster=w588, "M2 ShutDown Command"=w589) -> (w587:T2)
                }
                frame "dbControl.bInstrumentShutDownCommand" {
                  n210 = Variant To Data(error in=w598, type=FALSE, Variant=w600) -> (data=w596:bool, error out=w597:errorcluster)
                  n211 = Bundle By Name(cluster=w595, "Instrument ShutDown Command"=w596) -> (w594:T2)
                }
                frame "dbControl.iControlMode" {
                  n212 = Variant To Data(error in=w605, type=u16 0, Variant=w606) -> (data=→"Control Mode 2":u16, error out=w604:errorcluster)
                }
              }
            }
            "?" <- w507
          }
          event "Reset Commands Main2": Value Change {
            # "5."
            n213 = event-data() -> ("NewVal"=w609:bool)  [unwired: 1 in, 3 out]
            n214 = case shown="True" w609 {
              tunnel: w619 -> [_ w624]
              tunnel: [_ w623] -> w614
              tunnel: [FALSE TRUE] -> w610
              frame False {
              }
              frame True {
                n215 = Index Array(array=w624, index=12) -> (element=w623:string)
              }
            }
            n216 = To Variant(anything=w610) -> (Variant=w615:variant)
            n217 = Bundle By Name(cluster=T4 {"node ID"="", "value"=variant, "timestamp (current time)"=timestamp(0 s since 1904-01-01), "node status"=0} ("request"), "node ID"=w614, "value"=w615) -> (w618:T4)
            n218 = Build Array(w618) -> (w617:T4[])
            n219 = call-poly <vilib>:"Multiple Write.vi"("error in (no error)"=w608, "requests"=w617, "OPC UA client refnum in"=w612) -> ("error out"=w607:errorcluster, "OPC UA client refnum out"=w613:T3)  [unwired: 5 in, 2 out]
          }
          event "Reset Alarms Main2": Value Change {
            # "5."
            n220 = event-data() -> ("NewVal"=w629:bool)  [unwired: 1 in, 3 out]
            n221 = case shown="True" w629 {
              tunnel: w630 -> [_ w642]
              tunnel: [_ w641] -> w628
              tunnel: [FALSE TRUE] -> w627
              frame False {
              }
              frame True {
                n222 = Index Array(array=w642, index=13) -> (element=w641:string)
              }
            }
            n223 = To Variant(anything=w627) -> (Variant=w634:variant)
            n224 = Bundle By Name(cluster=T4 {"node ID"="", "value"=variant, "timestamp (current time)"=timestamp(0 s since 1904-01-01), "node status"=0} ("request"), "node ID"=w628, "value"=w634) -> (w637:T4)
            n225 = Build Array(w637) -> (w636:T4[])
            n226 = call-poly <vilib>:"Multiple Write.vi"("error in (no error)"=w626, "requests"=w636, "OPC UA client refnum in"=w632) -> ("error out"=w625:errorcluster, "OPC UA client refnum out"=w633:T3)  [unwired: 5 in, 2 out]
          }
        }
        n227 = local read "stop"() -> (w497:bool)
        n228 = Or(x=w498, y=w497) -> (x .or. y?=w503:bool)
      }
      n229 = call <vilib>:"Delete Monitored Nodes.vi"("error in (no error)"=w41, "node IDs"=w17, "subscription ID in"=w35, "OPC UA client refnum in"=w42) -> ("error out"=w39:errorcluster, "OPC UA client refnum out"=w40:T3)  [unwired: 3 in, 3 out]
      n230 = call <vilib>:"Delete Monitored Nodes.vi"("error in (no error)"=w13, "node IDs"=w4, "subscription ID in"=w28, "OPC UA client refnum in"=w14) -> ()  [unwired: 3 in, 5 out]
      n231 = call <vilib>:"Delete Monitored Nodes.vi"("error in (no error)"=w7, "node IDs"=w3, "subscription ID in"=w22, "OPC UA client refnum in"=w8) -> ()  [unwired: 3 in, 5 out]
      n232 = Build Array(w35, w28, w22) -> (w34:T7[])
      n233 = call <vilib>:"Delete Subscriptions.vi"("error in (no error)"=w39, "subscription IDs"=w34, "OPC UA client refnum in"=w40) -> ("error out"=w37:errorcluster, "OPC UA client refnum out"=w38:T3)  [unwired: 6 in, 1 out]
      n234 = call <vilib>:"Disconnect.vi"("error in (no error)"=w37, "OPC UA client refnum in"=w38) -> ("error out"=w32:errorcluster)  [unwired: 9 in]
      n235 = call <vilib>:"Simple Error Handler.vi"("error in (no error)"=w32) -> ()  [unwired: 4 in, 5 out]
    }
    frame Error {
      n236 = Unbundle By Name(w790) -> ("code"=w789:i32)
      n237 = case shown="-356612" w789 {
        frame 0, Default {
        }
        frame -356612 {
          n238 = One Button Dialog(message="A communication problem occurred. Ensure that the OPC UA server that you specify in the server endpoint URL is running and the network between the OPC UA server and the OPC UA client is connectable.") -> ()  [unwired: 1 in, 1 out]
        }
      }
    }
  }
